vi "EjemploTanque.vi"() -> ()   [LabVIEW 2020]
panel:
  out "Nivel Medio":bool
  in  "Nivel Medio":dbl
  in  "Set Point Nivel Bajo":dbl=10.0
  in  "Set Point Nivel Alto":dbl=90.0
  out "Iteraciones":i32
  in  "stop":bool
  out "Nivel Bajo":bool
  out "Nivel Alto":bool
  out "Waveform Chart":dbl(graph)
  in  "Dial":dbl(knob) scale=0.0..100.0
  out "Tank":dbl(slide) scale=0.0..100.0
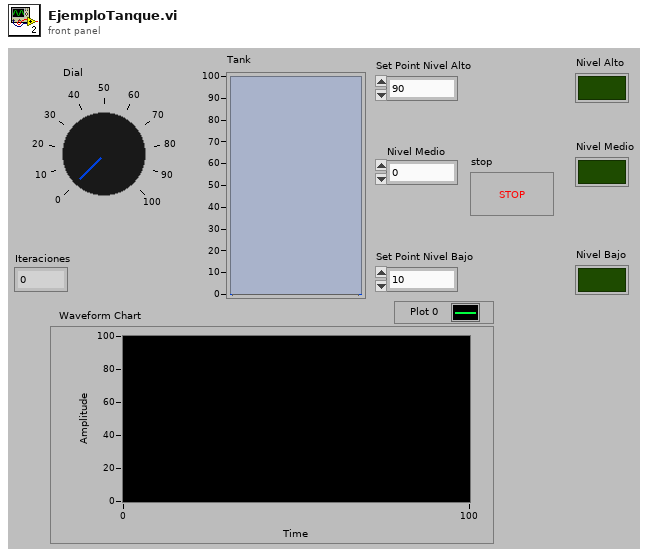
[diagram p1: front panel]
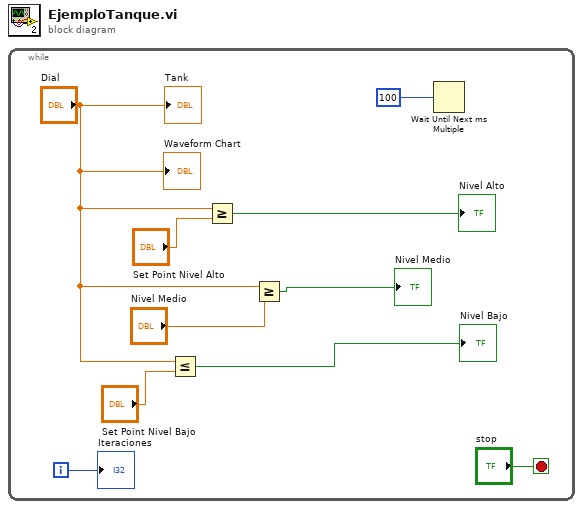
[diagram p0: block diagram]
diagram:
  n1 = while {
    i -> [w7]
    stop <- "stop" stop-if-true
    n2 = Less Or Equal?(x="Dial", y="Set Point Nivel Bajo") -> (x <= y?=→"Nivel Bajo":bool)
    n3 = Greater Or Equal?(x="Dial", y="Set Point Nivel Alto") -> (x >= y?=→"Nivel Alto":bool)
    n4 = Greater Or Equal?(x="Dial", y="Nivel Medio") -> (x >= y?=→"Nivel Medio":bool)
    n5 = Wait Until Next ms Multiple(millisecond multiple=u32 100) -> ()  [unwired: 1 out]
    "Tank" <- "Dial"
    "Waveform Chart" <- "Dial"
    "Iteraciones" <- w7
  }
